vi "FitnessOnTrainData.vi"(1 "Init? (F)":bool, 2 "Data":variant, 3 "Phenotype":i32[](array[numeric])) -> (0 "Fitness":dbl)   [LabVIEW 2016, in "Optimal Frequency Bands Search.lvlib" / "GeneticAlgorithm.lvlib"]
doc: "Расчет функции приспособленности для особи. При расчете приспособленности классификатор на основе многослойного персептрона обучается и тестируется на обучающих данных."
uses:
  GeneticAlgorithm.lvlib
  _vlib/OptFreqBandsSearch.lvclass
  _vlib/OFBS_DataTypes.ctl
  Optimal Frequency Bands Search.lvlib
panel:
  # "This VI is a part of BCI Design library, http://www.ru-bci.org \nCopyright © 2020, Sotnikov Peter, All rights reserved. License: GNU GPLv3"
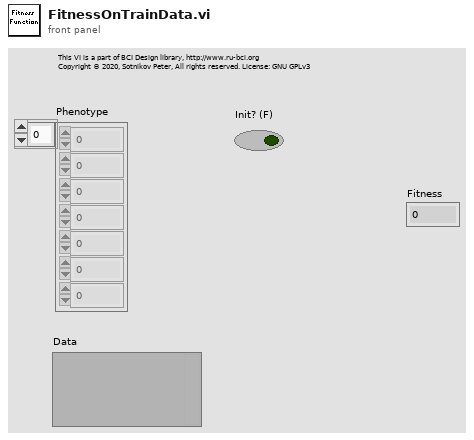
[diagram p1: front panel]
types:
  T1 = typedef "Optimal Frequency Bands Search.lvlib/OFBS_DataTypes.ctl" = enum16{"Training Data", "Test Data", "Training Data (cross-check)", "Test Data (cross-check)"}
  T2 = typedef "Optimal Frequency Bands Search.lvlib/OFBS_ClassifierTypes.ctl" = enum16{"Multilayer perceptron", "k NN Classifier", "SVM Committee", "Mahalanobis distance", "SVM Classifier"}
  T3 = typedef "NILabs_MLT.lvlib/ml_BP_Project.ctl" = cluster{"Training Data":T4, "Normalize Info":T5, "3-layer NN":T6, "Ternimal Condition":T7}
  T4 = typedef "NILabs_MLT.lvlib/ml_BP_Data.ctl" = cluster{"dim in":i32, "dim out":i32, "# samples":i32, "Input":dbl[][], "Output":dbl[][]}
  T5 = typedef "NILabs_MLT.lvlib/ml_BP_Normalize Data.ctl" = cluster{"input min":dbl[], "input max":dbl[], "output min":dbl[], "output max":dbl[]}
  T6 = typedef "NILabs_MLT.lvlib/ml_BP_3layer Feedforward.ctl" = cluster{"# input neuron ":i32, "# hidden neuron":i32, "# output neuron":i32, "Weight (I->H)":dbl[][], "Weight (H->O)":dbl[][], "Output":dbl[][], "Hidden Out":dbl[][], "Derivation Output":dbl[][], "Derivation Hidden":dbl[][], "dw (I->H)":dbl[][], "dw (H->O)":dbl[][]}
  T7 = typedef "NILabs_MLT.lvlib/ml_BP_Terminal Condition.ctl" = cluster{"min MSE":dbl, "min delta MSE":dbl, "min step length":dbl, "max iteration":dbl}
  T8 = typedef "IMAQ Classifier Session.ctl" = refnum<k1>
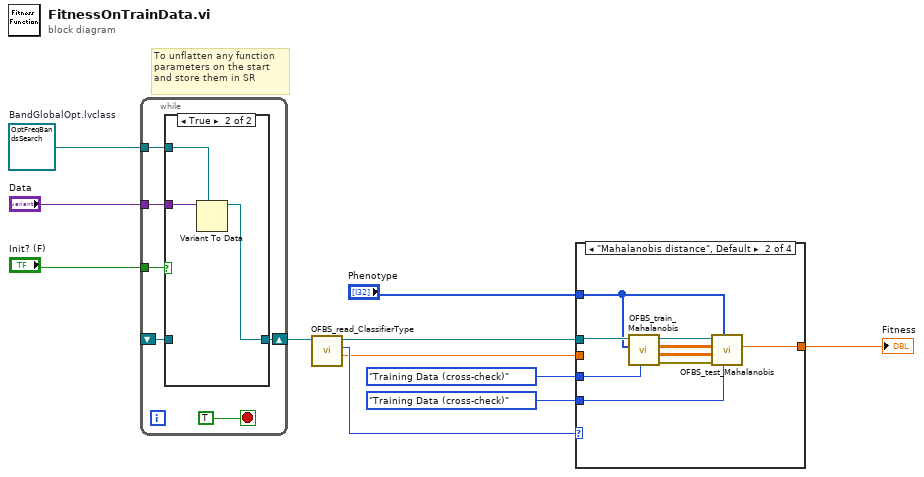
[diagram p0: block diagram]
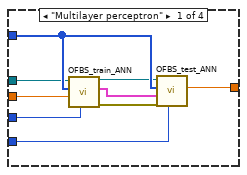
[diagram p2: hidden frame]
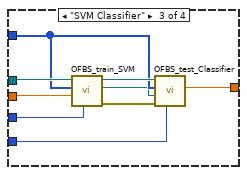
[diagram p3: hidden frame]
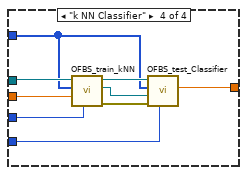
[diagram p4: hidden frame]
diagram:
  w9 = refnum<class "OptFreqBandsSearch.lvclass"> refnum  # BandGlobalOpt.lvclass
  # "To unflatten any function\nparameters on the start\nand store them in SR"
  n1 = while {
    tunnel: "Data" -> [w15]
    tunnel: "Init? (F)" -> [w16]
    shift-right: [w14] -> w7
    shift-left: _ -> [w13]
    tunnel: w9 -> [w12]
    stop <- TRUE stop-if-true
    n2 = case shown="True" w16 {
      tunnel: w15 -> [_ w21]
      tunnel: [w18 w19] -> w14
      tunnel: w13 -> [w18 _]
      tunnel: w12 -> [_ w20]
      frame False {
      }
      frame True {
        n3 = Variant To Data(type=w20, Variant=w21) -> (data=w19:refnum<class "OptFreqBandsSearch.lvclass">)  [unwired: 1 in, 1 out]
      }
    }
  }
  n4 = call-dynamic "OFBS_read_ClassifierType.vi"("OptFreqBandsSearch in"=w7) -> ("Classifier Metaparameter"=w1:dbl, "ClassifierType"=w3:T2, "OptFreqBandsSearch out"=w5:refnum<class "OptFreqBandsSearch.lvclass">)  [unwired: 7 in, 1 out]
  n5 = case shown="\"Mahalanobis distance\", Default" w3 {
    tunnel: [w30 w32 w41 w52] -> w2
    tunnel: "Phenotype" -> [w29 w37 w45 w53]
    tunnel: w5 -> [w25 w39 w48 w57]
    tunnel: OFBS_DataTypes."Training Data (cross-check)" ("DataType") -> [w24 w33 w44 w51]
    tunnel: OFBS_DataTypes."Training Data (cross-check)" ("DataType") -> [w23 w31 w43 w50]
    tunnel: w1 -> [w22 _ w40 w49]
    frame "Multilayer perceptron" {
      n6 = call "OFBS_train_ANN.vi"("Train Data"=w24, "# of hidden neurons"=w22, "Parameters"=w29, "OFBS class in"=w25) -> ("error out"=w26:errorcluster, "ANN out"=w27:T3, "OFBS class out"=w28:refnum<class "OptFreqBandsSearch.lvclass">)  [unwired: 4 in, 1 out]
      n7 = call "OFBS_test_ANN.vi"("Test Data"=w23, "error in (no error)"=w26, "ANN in"=w27, "Parameters"=w29, "OFBS class in"=w28) -> ("Accuracy"=w30:dbl)  [unwired: 3 in, 3 out]
    }
    frame "Mahalanobis distance", Default {
      n8 = call "OFBS_train_Mahalanobis.vi"("Train Data"=w33, "Parameters"=w37, "OFBS class in"=w39) -> ("error out"=w34:errorcluster, "Mean vectors"=w35:dbl[][], "Covariance matricies (inversed)"=w36:dbl[][][], "OFBS class out"=w38:refnum<class "OptFreqBandsSearch.lvclass">)  [unwired: 5 in]
      n9 = call "OFBS_test_Mahalanobis.vi"("Test Data"=w31, "Parameters"=w37, "error in (no error)"=w34, "Mean vectors"=w35, "Covariance matricies (inversed)"=w36, "OFBS class in"=w38) -> ("Accuracy"=w32:dbl)  [unwired: 2 in, 3 out]
    }
    frame "SVM Classifier" {
      n10 = call "OFBS_train_SVM.vi"("Train Data"=w44, "Nu"=w40, "Parameters"=w45, "OFBS class in"=w48) -> ("error out"=w46:errorcluster, "Classifier Session (out)"=w42:T8, "OFBS class out"=w47:refnum<class "OptFreqBandsSearch.lvclass">)  [unwired: 4 in, 1 out]
      n11 = call "OFBS_test_Classifier.vi"("Test Data"=w43, "error in (no error)"=w46, "Classifier Session"=w42, "Parameters"=w45, "OFBS class in"=w47) -> ("Accuracy"=w41:dbl)  [unwired: 3 in, 3 out]
    }
    frame "k NN Classifier" {
      n12 = call "OFBS_train_kNN.vi"("Train Data"=w51, "k"=w49, "Parameters"=w53, "OFBS class in"=w57) -> ("error out"=w55:errorcluster, "Classifier Session (out)"=w54:T8, "OFBS class out"=w56:refnum<class "OptFreqBandsSearch.lvclass">)  [unwired: 4 in, 1 out]
      n13 = call "OFBS_test_Classifier.vi"("Test Data"=w50, "error in (no error)"=w55, "Classifier Session"=w54, "Parameters"=w53, "OFBS class in"=w56) -> ("Accuracy"=w52:dbl)  [unwired: 3 in, 3 out]
    }
  }
  "Fitness" <- w2
